vi "Set Params.vi"(8 "error in (no error)":errorcluster, 10 "Search Params":T1, 11 "Search in":refnum<class "Search.lvclass">) -> (0 "error out":errorcluster, 3 "Search out":refnum<class "Search.lvclass">)   [LabVIEW 2020, in "Better Search.lvlib" / "Search.lvclass"]
uses:
  Search.lvclass
  Data Types/Search Params.ctl
  Data Types/Search Type.ctl
  Data Types/Search Scope.ctl
  Data Types/Scope Options.ctl
  Search.lvclass/Search.ctl
  Better Search.lvlib
panel:
  # "Exclude"
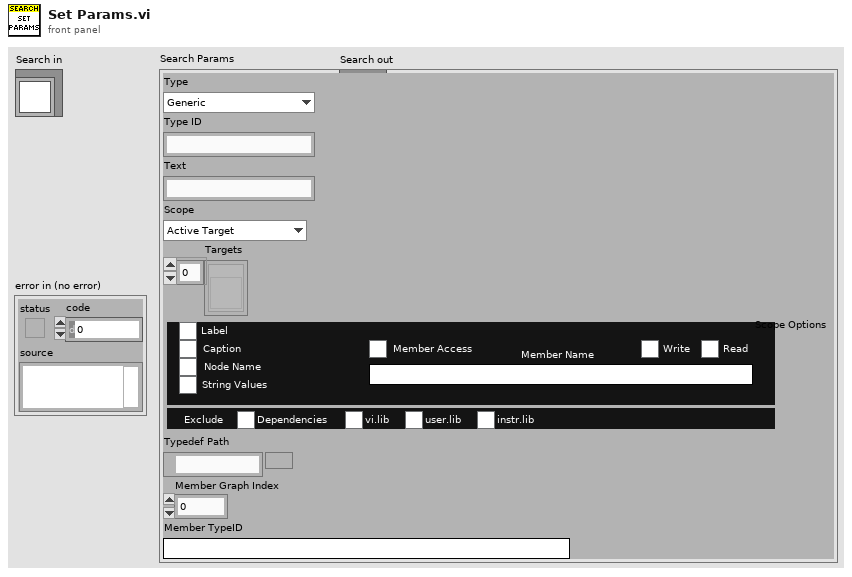
[diagram p1: front panel]
types:
  T1 = typedef "Better Search.lvlib/Search Params.ctl" = cluster{"Type":T2, "Type ID":string, "Text":string, "Scope":T3, "Targets":refnum<vi>[], "Scope Options":T4, "Typedef Path":path, "Member Graph Index":i32, "Member TypeID":string}
  T2 = typedef "Better Search.lvlib/Search Type.ctl" = enum16{"Generic", "Text", "Data Type", "VI", "Node"}
  T3 = typedef "Better Search.lvlib/Search Scope.ctl" = enum16{"Active Target", "Active Project", "Specific Targets", "Active VI", "Active Hierarchy"}
  T4 = typedef "Better Search.lvlib/Scope Options.ctl" = cluster{"Include Labels":bool, "Include Captions":bool, "Include Node Name":bool, "Member Access":bool, "Member Read":bool, "Member Write":bool, "Member Name":string, "String Value":bool, "Dependencies":bool, "vi.lib":bool, "user.lib":bool, "instr.lib":bool}
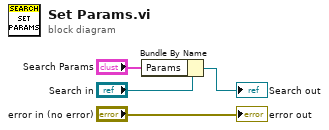
[diagram p0: block diagram]
diagram:
  n1 = Bundle By Name(cluster="Search in", "Params"="Search Params") -> (→"Search out":refnum<class "Search.lvclass">)
  "error out" <- "error in (no error)"
